vi "CLSUIP_GrowthFactor.vi"(1 "Terminals as icons":bool, 2 "Number of terminals":i32) -> (0 "Multiplication Factor":cluster{"Left":i32, "Top":i32})   [LabVIEW 2021, in "MemberVICreation.lvlib"]
uses:
  <resource>/Framework/Providers/LVClassLibrary/NewAccessors/MemberVICreation.lvlib
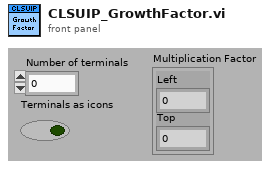
[diagram p1: front panel]
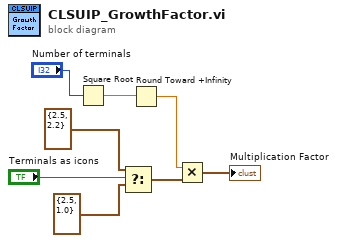
[diagram p0: block diagram]
diagram:
  n1 = Square Root(x="Number of terminals") -> (sqrt(x)=w5:dbl)
  n2 = Select(t=cluster{"Left":dbl, "Top":dbl} {"Left"=2.5, "Top"=2.2} ("Multiplication Factor"), s="Terminals as icons", f=cluster{"Left":dbl, "Top":dbl} {"Left"=2.5, "Top"=1.0} ("Multiplication Factor")) -> (s? t:f=w4:cluster{"Left":dbl, "Top":dbl})
  n3 = Round Toward +Infinity(x=w5) -> (ceil(x): smallest int >= x=w3:dbl)
  n4 = Multiply(x=w3, y=w4) -> (x*y=→"Multiplication Factor":cluster{"Left":dbl, "Top":dbl})
